vi "H036 Harsh Pandit SCADA Lab 8b Sem 6.vi"() -> ()   [LabVIEW 2018]
panel:
  out "Number":dbl
  in  "Expression to be found":string
  in  "Array":string[](array[string])
  # "Experiment 8B: Build a VI which finds the number of occurences of particular string in array\nof strings"
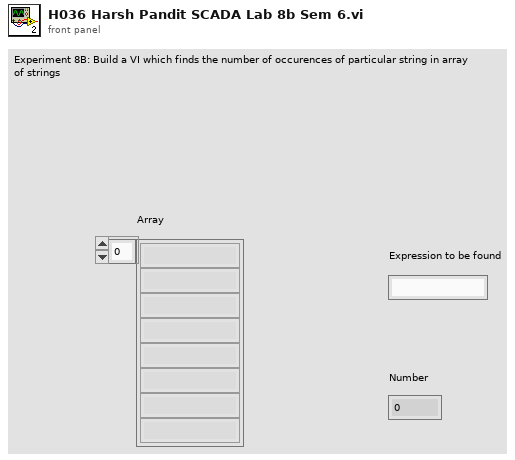
[diagram p1: front panel]
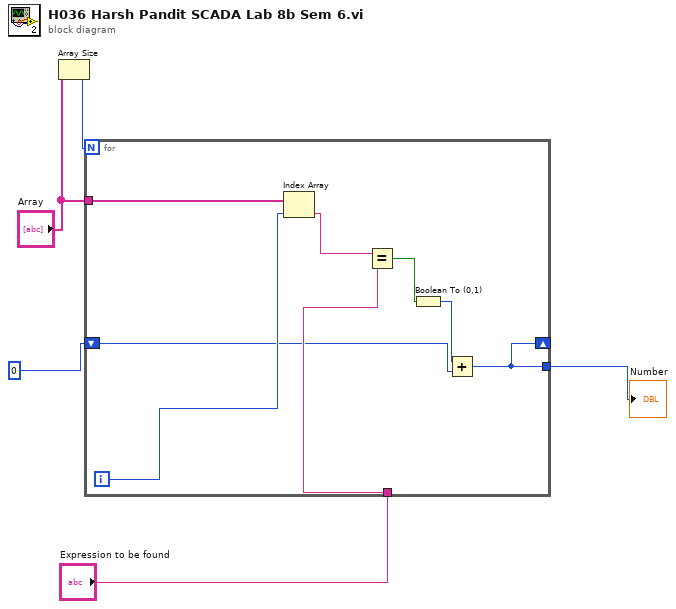
[diagram p0: block diagram]
diagram:
  n1 = Array Size(array="Array") -> (size(s)=w4:i32)
  n2 = for {
    N: w4 -> [_]
    tunnel: "Array" -> [w13]
    tunnel: "Expression to be found" -> [w10]
    shift-right: [w6] -> _
    shift-left: 0 -> [w7]
    tunnel: [w6] -> w1
    i -> [w12]
    n3 = Index Array(array=w13, index=w12) -> (element=w11:string)
    n4 = Equal?(x=w11, y=w10) -> (x = y?=w9:bool)
    n5 = Boolean To (0,1)(Boolean=w9) -> (0, 1=w8:i16)
    n6 = Add(x=w8, y=w7) -> (x+y=w6:i32)
  }
  "Number" <- w1
